vi "create.AddOrderExpanded.vi"(11 "AddOrderExpanded.Parameters":T1={"Time Offset"=447000, "Order Id"="ORID0001", "Quantity"=20000, "Symbol"="AAPL", "Side Indicator"="B", "Price"=0.905, "Participant Id"="B", "Customer Indicator"="B"}) -> (2 "Bytes.Out":u8[](array[numeric])=[34, 33, 24, 210, 6, 0, 79, 82, 73, 68, 48, 48, 48, 49, 66, 32, 78, 0, 0, 65, 65, 80, 76, 32, 32, 90, 35, 0, 0, 0, 0, 0, 0, 1] format="%.0x", 3 "MessageBase out":refnum<class "AddOrderExpanded.lvclass">)   [LabVIEW 2022 SP3]
uses:
  AddOrder/AddOrderExpanded.Parameters.ctl
  AddOrder/AddOrderExpanded.lvclass
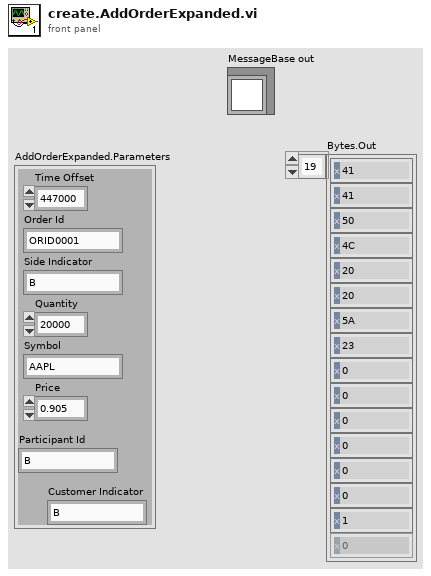
[diagram p1: front panel]
types:
  T1 = typedef "AddOrderExpanded.lvclass/AddOrderExpanded.Parameters.ctl" = cluster{"Time Offset":u32, "Order Id":string, "Quantity":u32, "Symbol":string, "Side Indicator":string, "Price":dbl, "Participant Id":string, "Customer Indicator":string}
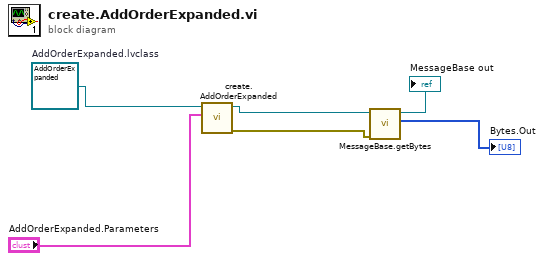
[diagram p0: block diagram]
diagram:
  w5 = refnum<class "AddOrderExpanded.lvclass"> refnum  # AddOrderExpanded.lvclass
  n1 = call-dynamic "create.AddOrderExpanded.vi"("AddOrderExpanded.Parameters"="AddOrderExpanded.Parameters", "AddOrderTest in"=w5) -> ("error out"=w2:errorcluster, "AddOrderTest out"=w4:refnum<class "AddOrderExpanded.lvclass">)  [unwired: 8 in]
  n2 = call-dynamic "MessageBase.getBytes.vi"("error in (no error)"=w2, "MessageBase in"=w4) -> ("Bytes.out"=→"Bytes.Out":u8[], "MessageBase out"=→"MessageBase out":refnum<class "AddOrderExpanded.lvclass">)  [unwired: 7 in, 1 out]
